vi "Memory.Pointer.Error Handling.Write Range to Error.vi"(7 "parameter":T1, 8 "value":u64, 9 "offset":i32, 10 "error in":errorcluster, 11 "pointer in":refnum<class "Memory.Pointer.lvclass">) -> (1 "new offset":i32, 2 "error out":errorcluster, 3 "pointer out":refnum<class "Memory.Pointer.lvclass">)   [LabVIEW 2016, in "Memory Manager.lvlib" / "Memory.Pointer.lvclass"]
uses:
  Memory.Pointer.lvclass
  Pointer.Void/Typedefs/Memory.Pointer.Parameters.ctl
  Memory.Pointer.lvclass/Memory.Pointer.ctl
  <vilib>/NI/Static Error Handling/VIs/Static Error Handling.Source Buffer.Write.Numeric.Scalar.Base10 (U64).vi
  <vilib>/NI/Static Error Handling/Static Error Handling.lvlib
  Pointer.Void/Memory.Pointer.Void.lvclass
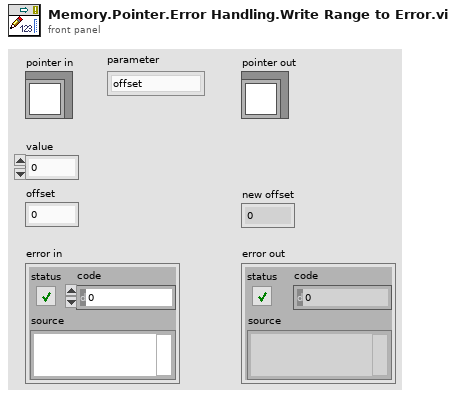
[diagram p1: front panel]
types:
  T1 = typedef "Memory Manager.lvlib/Memory.Pointer.Void.lvclass/Memory.Pointer.Parameters.ctl" = enum16{"offset", "length", "size", "subset"}
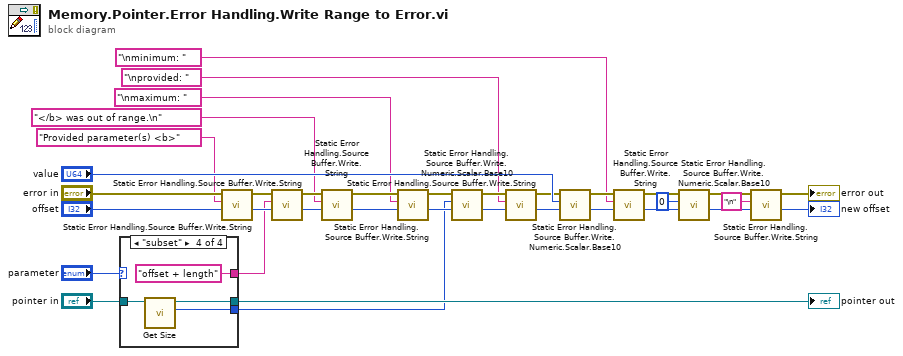
[diagram p0: block diagram]
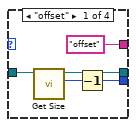
[diagram p2: hidden frame]
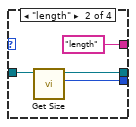
[diagram p3: hidden frame]
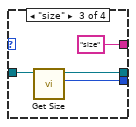
[diagram p4: hidden frame]
diagram:
  n1 = case shown="\"subset\"" "parameter" {
    tunnel: "pointer in" -> [w39 w43 w47 w51]
    tunnel: ["offset" "length" "size" "offset + length"] -> w5
    tunnel: [w36 w42 w46 w50] -> w2
    tunnel: [w37 w41 w45 w49] -> w29
    frame "offset" {
      n2 = call "Get Size.vi"("Pointer in"=w39) -> ("size"=w38:u64, "Pointer out"=w37:refnum<class "Memory.Pointer.lvclass">)  [unwired: 8 in, 1 out]
      n3 = Decrement(x=w38) -> (x-1=w36:u64)
    }
    frame "length" {
      n4 = call "Get Size.vi"("Pointer in"=w43) -> ("size"=w42:u64, "Pointer out"=w41:refnum<class "Memory.Pointer.lvclass">)  [unwired: 8 in, 1 out]
    }
    frame "size" {
      n5 = call "Get Size.vi"("Pointer in"=w47) -> ("size"=w46:u64, "Pointer out"=w45:refnum<class "Memory.Pointer.lvclass">)  [unwired: 8 in, 1 out]
    }
    frame "subset" {
      n6 = call "Get Size.vi"("Pointer in"=w51) -> ("size"=w50:u64, "Pointer out"=w49:refnum<class "Memory.Pointer.lvclass">)  [unwired: 8 in, 1 out]
    }
  }
  "pointer out" <- w29
  n7 = call <vilib>:"Static Error Handling.Source Buffer.Write.String.vi"("offset"="offset", "string"="Provided parameter(s) <b>", "error in"="error in") -> ("new offset"=w10:i32, "error out"=w12:errorcluster)  [unwired: 7 in]
  n8 = call <vilib>:"Static Error Handling.Source Buffer.Write.String.vi"("offset"=w10, "string"=w5, "error in"=w12) -> ("new offset"=w9:i32, "error out"=w11:errorcluster)  [unwired: 7 in]
  n9 = call <vilib>:"Static Error Handling.Source Buffer.Write.String.vi"("offset"=w9, "string"="</b> was out of range.\n", "error in"=w11) -> ("new offset"=w8:i32, "error out"=w7:errorcluster)  [unwired: 7 in]
  n10 = call <vilib>:"Static Error Handling.Source Buffer.Write.String.vi"("offset"=w8, "string"="\nmaximum: ", "error in"=w7) -> ("new offset"=w24:i32, "error out"=w27:errorcluster)  [unwired: 7 in]
  n11 = call-poly <vilib>:"Static Error Handling.Source Buffer.Write.Numeric.Scalar.Base10.vi"("offset"=w24, "value"=w2, "error in"=w27) -> ("new offset"=w25:i32, "error out"=w26:errorcluster)  [unwired: 7 in]
  n12 = call <vilib>:"Static Error Handling.Source Buffer.Write.String.vi"("offset"=w25, "string"="\nprovided: ", "error in"=w26) -> ("new offset"=w21:i32, "error out"=w22:errorcluster)  [unwired: 7 in]
  n13 = call-poly <vilib>:"Static Error Handling.Source Buffer.Write.Numeric.Scalar.Base10.vi"("offset"=w21, "value"="value", "error in"=w22) -> ("new offset"=w19:i32, "error out"=w20:errorcluster)  [unwired: 7 in]
  n14 = call <vilib>:"Static Error Handling.Source Buffer.Write.String.vi"("offset"=w19, "string"="\nminimum: ", "error in"=w20) -> ("new offset"=w17:i32, "error out"=w18:errorcluster)  [unwired: 7 in]
  n15 = call-poly <vilib>:"Static Error Handling.Source Buffer.Write.Numeric.Scalar.Base10.vi"("offset"=w17, "value"=u64 0 ("size"), "error in"=w18) -> ("new offset"=w14:i32, "error out"=w16:errorcluster)  [unwired: 7 in]
  n16 = call <vilib>:"Static Error Handling.Source Buffer.Write.String.vi"("offset"=w14, "string"="\n", "error in"=w16) -> ("new offset"=→"new offset":i32, "error out"=→"error out":errorcluster)  [unwired: 7 in]
